vi "Set EDS File Path.vi"(10 "EDS File Path":path, 11 "EDS in":refnum<class "EDS.lvclass">) -> (3 "EDS out":refnum<class "EDS.lvclass">)   [LabVIEW 2024, in "EDS.lvlib" / "EDS.lvclass"]
uses:
  EDS.lvclass
  EDS.lvclass/EDS.ctl
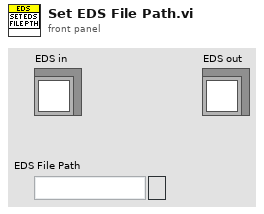
[diagram p1: front panel]
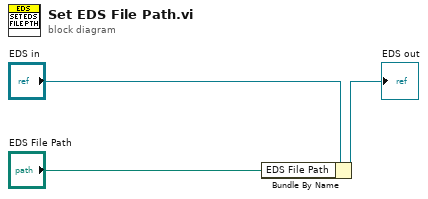
[diagram p0: block diagram]
diagram:
  n1 = Bundle By Name(cluster="EDS in", "EDS File Path"="EDS File Path") -> (→"EDS out":refnum<class "EDS.lvclass">)
